vi "REACTOR_STOP.vi"(9 "error in (no error)":errorcluster, 10 "Stop":enum16{"Continue", "Stop", "Default"}(ring)) -> (1 "error out":errorcluster, 2 "Stop?":bool)   [LabVIEW 2017]
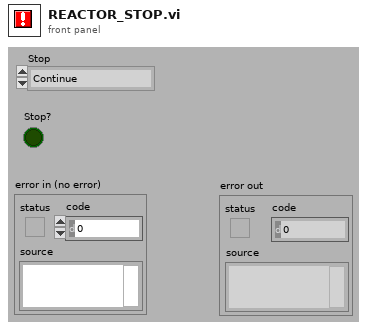
[diagram p1: front panel]
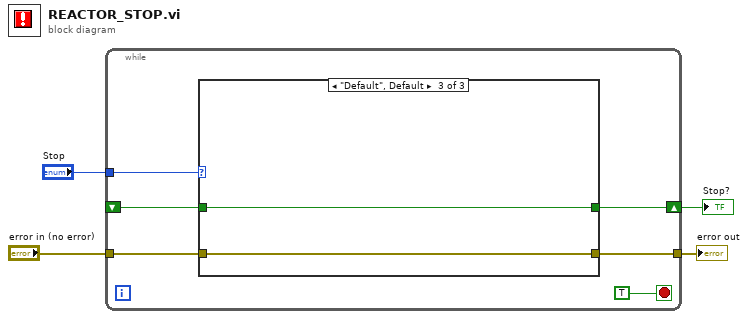
[diagram p0: block diagram]
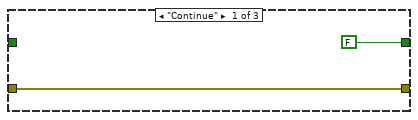
[diagram p2: hidden frame]
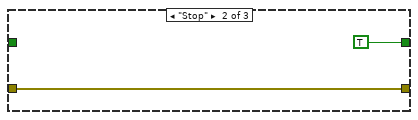
[diagram p3: hidden frame]
diagram:
  n1 = while {
    tunnel: "Stop" -> [w10]
    shift-right: [w8] -> w3
    shift-left: _ -> [w7]
    tunnel: "error in (no error)" -> [w6]
    tunnel: [w5] -> w1
    stop <- TRUE stop-if-true
    n2 = case shown="\"Default\", Default" w10 {
      tunnel: [FALSE TRUE w16] -> w8
      tunnel: w7 -> [_ _ w16]
      tunnel: w6 -> [w11 w13 w15]
      tunnel: [w11 w13 w15] -> w5
      frame "Continue" {
      }
      frame "Stop" {
      }
      frame "Default", Default {
      }
    }
  }
  "Stop?" <- w3
  "error out" <- w1
